vi "MMEM_STOR_CIT_FORM.vi"(0 "VISA IN":refnum<visa-resource-name>, 5 "error in":errorcluster, 7 "FileName":string) -> (14 "VISA Out":refnum<visa-resource-name>, 19 "error out":errorcluster)   [LabVIEW 2018, in "PNA-X.lvlib"]
doc: "MMEMory:STORe:CITifile:FORMat <filename> \n1613\n\n(Write only) Saves FORMATTED trace data to .cti file. Learn more. \nParameters \n<filename> Any drive and folder name that already exists. \nIf the same level as \"C:\\Program Files\\Agilent\\Network Analyzer\\Documents\", \nthen no punctuation is required \nMMEM:STOR:CIT:DATA MYFile \nIf the new folder is at a different level than \"C:\\Program Files\\Agilent\\Network \nAnalyzer\\Documents\", use a slash (\\) before the folder name and enclose in \nquotes. \nmmemory:cdirectory '\\automation' 'changes default directory up \none level. \nYou can use an absolute path to specify the new folder. \nmmemory:cdirectory 'c:\\automation\\service' \nQuery Syntax Not Applicable \nDefault C:\\Program Files\\Agilent\\Network Analyzer\\Documents'"
uses:
  PNA-X.lvlib
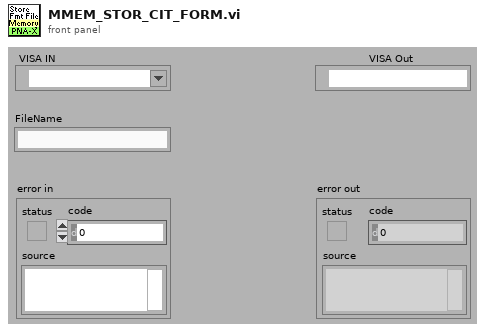
[diagram p1: front panel]
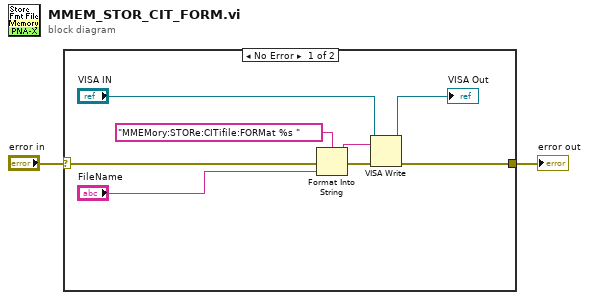
[diagram p0: block diagram]
diagram:
  n1 = case shown="No Error" "error in" {
    selector: "error in" -> [w10 w11]
    tunnel: [w5 w11] -> w1
    frame No Error {
      n2 = Format Into String(format string="MMEMory:STORe:CITifile:FORMat %s " ("Cmdline"), error in=w10, "FileName") -> (resulting string=w8:string, error out=w9:errorcluster)  [unwired: 1 in]
      n3 = VISA Write(VISA resource name="VISA IN", write buffer=w8, error in (no error)=w9) -> (VISA resource name out=→"VISA Out":refnum<visa-resource-name>, error out=w5:errorcluster)  [unwired: 1 out]
    }
    frame Error {
    }
  }
  "error out" <- w1
